vi "Load Palette Images.vi"(8 "error in (no error)":errorcluster, 11 "Palette Image Folder":path=path "C:/Users/FAST Lab/Perforce/john.pfisterer_AMRGROBJ07MYKD_5284/Pfizer/2018-1080 Pfizer FAST/Software/Images") -> (0 "error out":errorcluster, 1 "Cursor IDs":refnum<k1>[](array[refnum]), 2 "[Thumbnails]":T1[](array[typedef]), 3 "new picture":picture)   [LabVIEW 2018]
uses:
  Thumbnail Cluster.ctl
panel:
  out "filenames":string[](array[string])
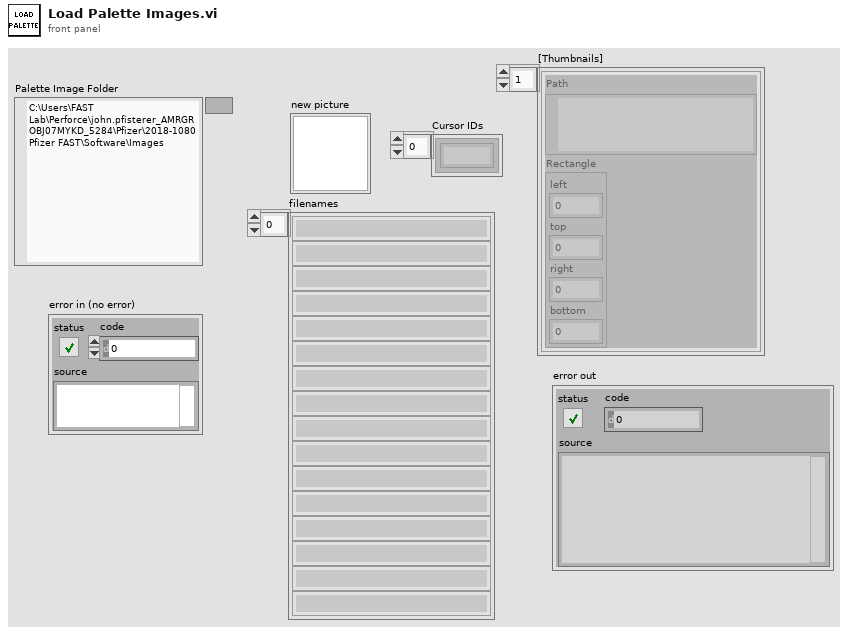
[diagram p1: front panel]
types:
  T1 = typedef "Thumbnail Cluster.ctl" = cluster{"Path":path, "Rectangle":cluster{"left":i16, "top":i16, "right":i16, "bottom":i16}}
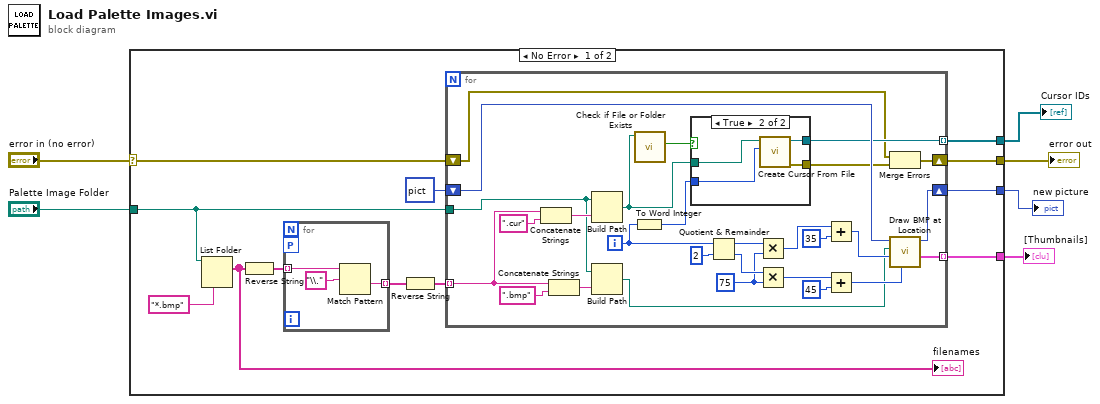
[diagram p0: block diagram]
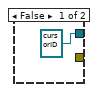
[diagram p2: hidden frame]
diagram:
  n1 = case shown="No Error" "error in (no error)" {
    selector: "error in (no error)" -> [w7 w55]
    tunnel: [w17 _] -> w6
    tunnel: "Palette Image Folder" -> [w16 _]
    tunnel: [w15 _] -> w4
    tunnel: [w9 _] -> w3
    tunnel: [w8 w55] -> w2
    frame No Error {
      n2 = List Folder(path=w16, pattern="*.bmp") -> (filenames=w13:string[])  [unwired: 2 in, 3 out]
      "filenames" <- w13
      n3 = Reverse String(1:w13) -> (0:w12:string[])
      n4 = for {
        tunnel: w12 -> [w21] mode=indexing
        tunnel: [w19] -> w11 mode=indexing
        workers-P: _ -> [_]
        n5 = Match Pattern(string=w21, regular expression="\\.") -> (after substring=w19:string)  [unwired: 1 in, 3 out]
      }
      n6 = Reverse String(1:w11) -> (0:w10:string[])
      n7 = for {
        tunnel: w16 -> [w31]
        shift-right: [w45] -> w17
        shift-left: picture data[5B] ("picture") -> [w46]
        tunnel: w10 -> [w30] mode=indexing
        tunnel: [w44] -> w15 mode=indexing
        tunnel: [w28] -> w9 mode=indexing
        shift-right: [w24] -> w8
        shift-left: w7 -> [w26]
        i -> [w27]
        w43 = 75 ("y")
        n8 = Concatenate Strings(w30, ".cur" ("string")) -> (w33:string)
        n9 = Concatenate Strings(w30, ".bmp" ("string")) -> (w35:string)
        n10 = Build Path(base path=w31, name or relative path=w33) -> (appended path=w23:path)
        n11 = Build Path(base path=w31, name or relative path=w35) -> (appended path=w36:path)
        n12 = To Word Integer(number=w27) -> (16bit integer=w29:i16)
        n13 = call <vilib>:"Check if File or Folder Exists.vi"("path"=w23) -> ("file or folder exists?"=w22:bool)  [unwired: 8 in, 2 out]
        n14 = case shown="True" w22 {
          tunnel: w23 -> [_ w54]
          tunnel: w29 -> [_ w53]
          tunnel: [refnum<k1> refnum ("cursor ID") w52] -> w28
          tunnel: [_ w51] -> w25
          frame False {
          }
          frame True {
            n15 = call <vilib>:"Create Cursor From File.vi"("cursor resource ID"=w53, "cursor file"=w54) -> ("error out"=w51:errorcluster, "cursor ID"=w52:refnum<k1>)  [unwired: 8 in]
          }
        }
        n16 = Quotient & Remainder(x=w27, y=2) -> (x-y*floor(x/y)=w47:i32, floor(x/y)=w48:i32)
        n17 = Multiply(x=w47, y=w43) -> (x*y=w42:i32)
        n18 = Multiply(x=w48, y=w43) -> (x*y=w40:i32)
        n19 = Add(x=w42, y=35) -> (x+y=w41:i32)
        n20 = Add(x=w40, y=45) -> (x+y=w39:i32)
        n21 = Merge Errors(w26, w25) -> (w24:errorcluster)
        n22 = call "Draw BMP at Location.vi"("top"=w39, "left"=w41, "selected path"=w36, "picture in"=w46) -> ("Thumbnail"=w44:T1, "picture out"=w45:picture)  [unwired: 5 in, 1 out]
      }
    }
    frame Error {
    }
  }
  "new picture" <- w6
  "[Thumbnails]" <- w4
  "Cursor IDs" <- w3
  "error out" <- w2
